vi "Read_Status.vi"() -> (0 "Water\n   (Lt)":dbl(slide) scale=0.0..10.0, 1 "Tea Powder\n       (Kg)":dbl(slide) scale=0.0..10.0, 2 "Coffee Powder\n         (Kg)":dbl(slide) scale=0.0..10.0, 3 "Milk\n (Lt)":dbl(slide) scale=0.0..10.0)   [LabVIEW 2014]
uses:
  <vilib>/Utility/file.llb/Read From Spreadsheet File (string).vi
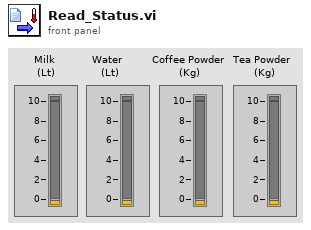
[diagram p1: front panel]
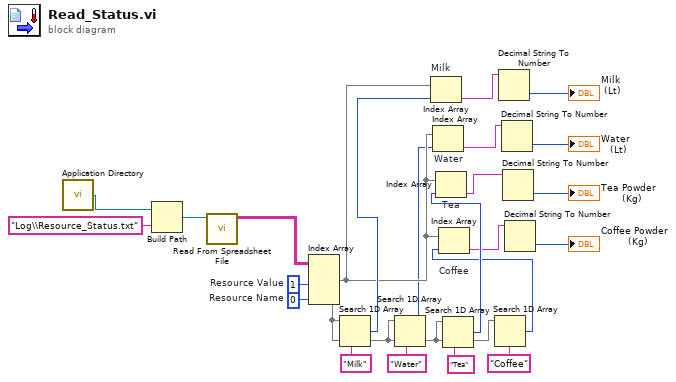
[diagram p0: block diagram]
diagram:
  w19 = 0  # Resource Name
  w20 = 1  # Resource Value
  n1 = call <vilib>:"Application Directory.vi"() -> ("Application Directory"=w24:path)
  n2 = Build Path(base path=w24, name or relative path="Log\\Resource_Status.txt") -> (appended path=w22:path)
  n3 = call-poly <vilib>:"Read From Spreadsheet File.vi"("file path (dialog if empty)"=w22) -> ("all rows"=w21:string[][])  [unwired: 6 in, 4 out]
  n4 = Index Array(array=w21, index (col) #1=w20, index (col) #2=w19) -> (element #1=w12:string[], element #2=w13:string[])  [unwired: 2 in]
  n5 = Search 1D Array(1D array=w13, element="Milk") -> (index of element=w14:i32)  [unwired: 1 in]
  n6 = Search 1D Array(1D array=w13, element="Water") -> (index of element=w11:i32)  [unwired: 1 in]
  n7 = Index Array "Milk"(array=w12, index=w14) -> (element=w7:string)
  n8 = Index Array "Water"(array=w12, index=w11) -> (element=w6:string)
  n9 = Search 1D Array(1D array=w13, element="Tea") -> (index of element=w10:i32)  [unwired: 1 in]
  n10 = Index Array "Tea"(array=w12, index=w10) -> (element=w5:string)
  n11 = Search 1D Array(1D array=w13, element="Coffee") -> (index of element=w9:i32)  [unwired: 1 in]
  n12 = Index Array "Coffee"(array=w12, index=w9) -> (element=w4:string)
  n13 = Decimal String To Number(string=w7) -> (number=→"Milk\n (Lt)":i32)  [unwired: 2 in, 1 out]
  n14 = Decimal String To Number(string=w6) -> (number=→"Water\n   (Lt)":i32)  [unwired: 2 in, 1 out]
  n15 = Decimal String To Number(string=w5) -> (number=→"Tea Powder\n       (Kg)":i32)  [unwired: 2 in, 1 out]
  n16 = Decimal String To Number(string=w4) -> (number=→"Coffee Powder\n         (Kg)":i32)  [unwired: 2 in, 1 out]
